vi "Set Select Event.vi"(8 "error in (no error)":errorcluster, 10 "Select Event":refnum<user-event>, 11 "DeviceArrayPanel in":refnum<class "DeviceArrayPanel.lvclass">) -> (0 "error out":errorcluster, 3 "DeviceArrayPanel out":refnum<class "DeviceArrayPanel.lvclass">)   [LabVIEW 2020, in "PicoG-App.lvlib" / "DeviceArrayPanel.lvclass"]
uses:
  DeviceArrayPanel.lvclass
  Device/Device.lvclass
  DeviceArrayPanel.lvclass/DeviceArrayPanel.ctl
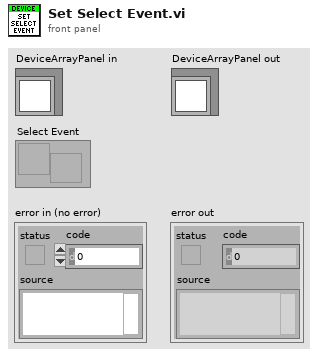
[diagram p1: front panel]
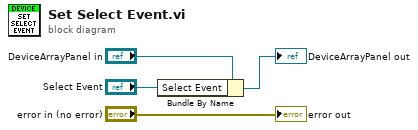
[diagram p0: block diagram]
diagram:
  n1 = Bundle By Name(cluster="DeviceArrayPanel in", "Select Event"="Select Event") -> (→"DeviceArrayPanel out":refnum<class "DeviceArrayPanel.lvclass">)
  "error out" <- "error in (no error)"
